vi "ep_Check Max Order Value.vi"(8 "error in (no error)":errorcluster, 11 "max sideband order":u8) -> (0 "error out":errorcluster)   [LabVIEW 2014, in "NI_EP_Motor Monitoring.lvlib"]
uses:
  <vilib>/addons/Electrical Power/Motor Monitoring/NI_EP_Motor Monitoring.lvlib
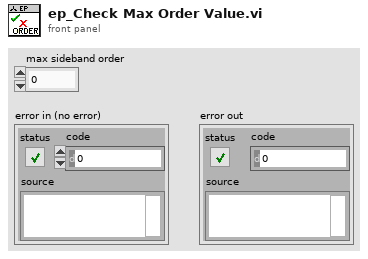
[diagram p1: front panel]
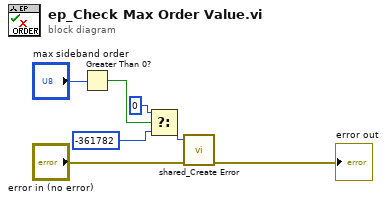
[diagram p0: block diagram]
diagram:
  n1 = Greater Than 0?(x="max sideband order") -> (x > 0?=w7:bool)
  n2 = Select(t=0 ("error code (0)"), s=w7, f=-361782 ("error code (0)")) -> (s? t:f=w2:i32)
  n3 = call <vilib>:"shared_Create Error.vi"("error in (no error)"="error in (no error)", "error code (0)"=w2) -> ("error out"=→"error out":errorcluster)  [unwired: 9 in]
